vi "powermeter-lambda.vi"(8 "error in (no error)":errorcluster, 10 "Lambda":dbl, 11 "PowerMeter":refnum<vi>) -> (0 "error out":errorcluster, 3 "Powermeter Out":refnum<vi>)   [LabVIEW 2016]
uses:
  controls/powermeter.ctl
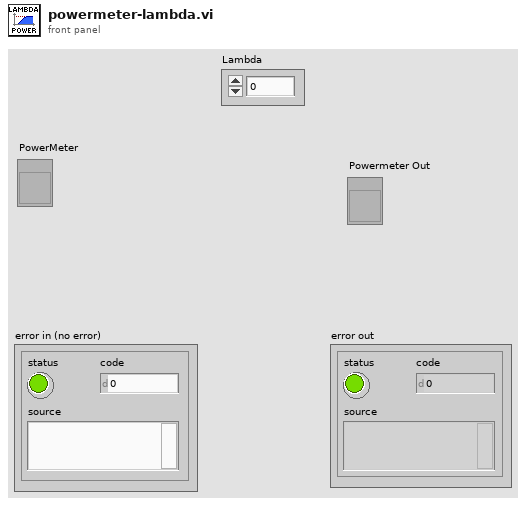
[diagram p1: front panel]
types:
  T1 = typedef "powermeter.ctl" = cluster{"Start":bool, "Serial ":string, "Model":string, "Sensor":string, "Power":dbl, "Density":bool, "Lambda":dbl, "Open":bool, "Save":bool, "reference":refnum<k7>, "hDevice":i32, "Dev. Std.":dbl, "Channel":i16}
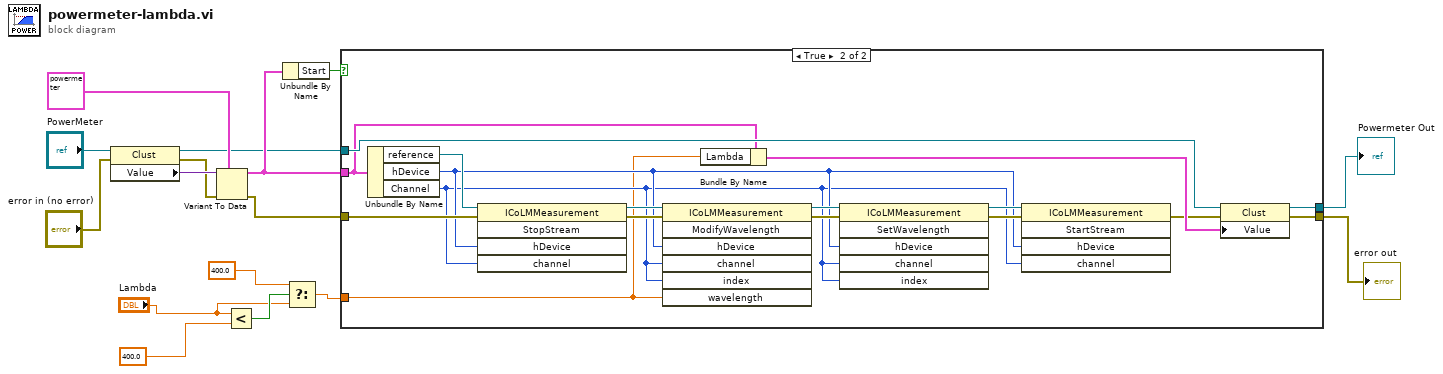
[diagram p0: block diagram]
diagram:
  n1 = property class="Clust"(reference="PowerMeter", error in="error in (no error)") -> (reference out=w7:refnum<vi>, error out=w11:errorcluster, "Value"=w12:variant)
  n2 = Variant To Data(error in=w11, type=T1 {"Start"=FALSE, "Serial "="", "Model"="", "Sensor"="", "Power"=0.0, "Density"=FALSE, "Lambda"=0.0, "Open"=FALSE, "Save"=FALSE, "reference"=refnum, "hDevice"=0, "Dev. Std."=0.0, "Channel"=0} ("Power Meter"), Variant=w12) -> (data=w9:T1, error out=w10:errorcluster)
  n3 = Less?(x="Lambda", y=400.0) -> (x < y?=w4:bool)
  n4 = Unbundle By Name(w9) -> ("Start"=w15:bool)
  n5 = Select(t=400.0, s=w4, f="Lambda") -> (s? t:f=w1:dbl)
  n6 = case shown="True" w15 {
    tunnel: w9 -> [_ w20]
    tunnel: w10 -> [w18 w34]
    tunnel: [w18 w23] -> w16
    tunnel: w7 -> [w17 w22]
    tunnel: [w17 w21] -> w6
    tunnel: w1 -> [_ w19]
    frame False {
    }
    frame True {
      n7 = Unbundle By Name(w20) -> ("reference"=w35:refnum<k7>, "hDevice"=w27:i32, "Channel"=w26:i16)
      n8 = invoke class="ICoLMMeasurement" method="StopStream"(reference=w35, error in=w34, "hDevice"=w27, "channel"=w26) -> (reference out=w32:refnum<k7>, error out=w33:errorcluster)  [unwired: 1 in, 3 out]
      n9 = invoke class="ICoLMMeasurement" method="ModifyWavelength"(reference=w32, error in=w33, "hDevice"=w27, "channel"=w26, "index"=w26, "wavelength"=w19) -> (reference out=w28:refnum<k7>, error out=w31:errorcluster)  [unwired: 1 in, 5 out]
      n10 = Bundle By Name(cluster=w20, "Lambda"=w19) -> (w25:T1)
      n11 = invoke class="ICoLMMeasurement" method="SetWavelength"(reference=w28, error in=w31, "hDevice"=w27, "channel"=w26, "index"=w26) -> (reference out=w30:refnum<k7>, error out=w29:errorcluster)  [unwired: 1 in, 4 out]
      n12 = invoke class="ICoLMMeasurement" method="StartStream"(reference=w30, error in=w29, "hDevice"=w27, "channel"=w26) -> (error out=w24:errorcluster)  [unwired: 1 in, 4 out]
      n13 = property class="Clust"(reference=w22, error in=w24, "Value"=w25) -> (reference out=w21:refnum<vi>, error out=w23:errorcluster)
    }
  }
  "error out" <- w16
  "Powermeter Out" <- w6
